vi "To bytes.vi"(3 "MsgPackString in":refnum<class "MsgPackString.lvclass">) -> (1 "Array":u8[](array[numeric]))   [LabVIEW 2020, in "MessagePack.lvlib" / "MsgPackString.lvclass"]
uses:
  MsgPackString.lvclass
  MsgPackString.lvclass/MsgPackString.ctl
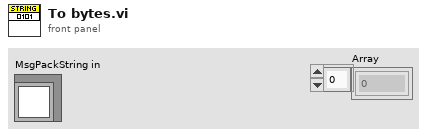
[diagram p1: front panel]
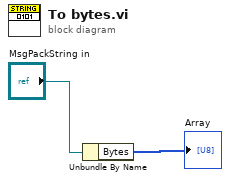
[diagram p0: block diagram]
diagram:
  n1 = Unbundle By Name("MsgPackString in") -> ("Bytes"=→"Array":u8[])
